vi "DTM Receiver Test.vi"() -> ()   [LabVIEW 2026, in "Nordic nRF52 DK DTM Test.lvlib"]
uses:
  Nordic nRF52 DK DTM Test.lvlib
  <vilib>/Analysis/1siggen.llb/Ramp Pattern by Delta.vi
  <vilib>/Analysis/NI_AALBase.lvlib
panel:
  in  "stop":bool
  out "Waveform Chart":T1(graph)
  out "iteration":i32
  out "Packets Received":u16
  out "Current Power":dbl
  out "Receiver Sensitivity, dBm":dbl
  in  "Baud Rate":u32=19200
  in  "Com Port Resource":refnum<visa-resource-name>="COM3"
  in  "Power Step, dBm":dbl=-0.2
  in  "Power Stop, dBm":dbl=-100.0
  in  "Power Start, dBm":dbl=-70.0
  in  "BLE Channel (0-39)":u8=19 max=39 step=1
  out "Rx Sens Threshold":i32
  in  "Packets to Generate":i32=1500
  in  "BLE Waveform Path":path=path "C:/git/LabVIEW_Bluetooth_Examples/BLE DTM Test/Waveform Files/BLE_PRBS9.tdms"
  in  "External Attenuation (dB)":dbl=1.1
  in  "Reference Clock Source":string(combo)="OnboardClock"
  in  "RFSG Resource":refnum<k15>="VST" caption="resource name"
  out "error out":errorcluster
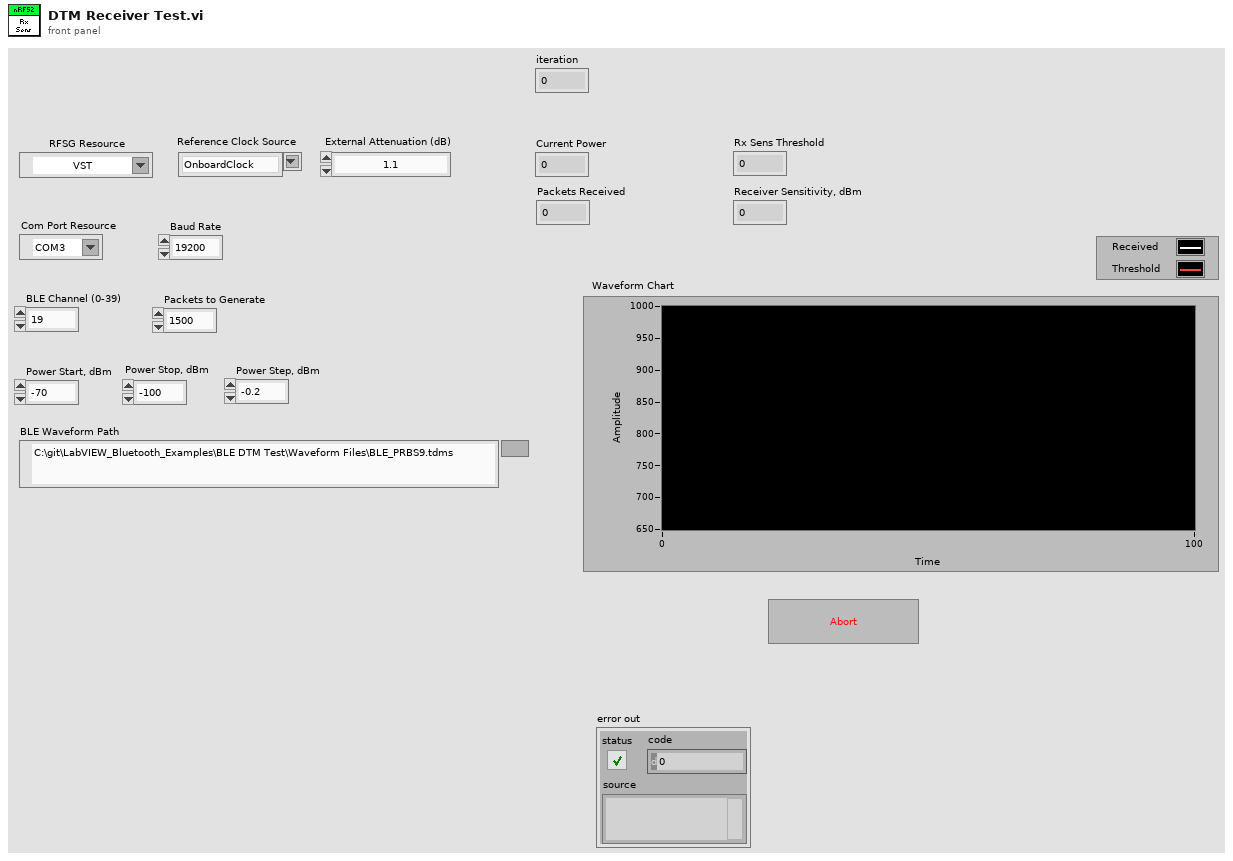
[diagram p1: front panel]
types:
  T1 = cluster{"Returned Packet Count":u16, "Rx Sensitivity Threshold":i32}
  T2 = cluster{"Returned Packet Count":u16, "Rx Sensitivity Threshold":i32}[]
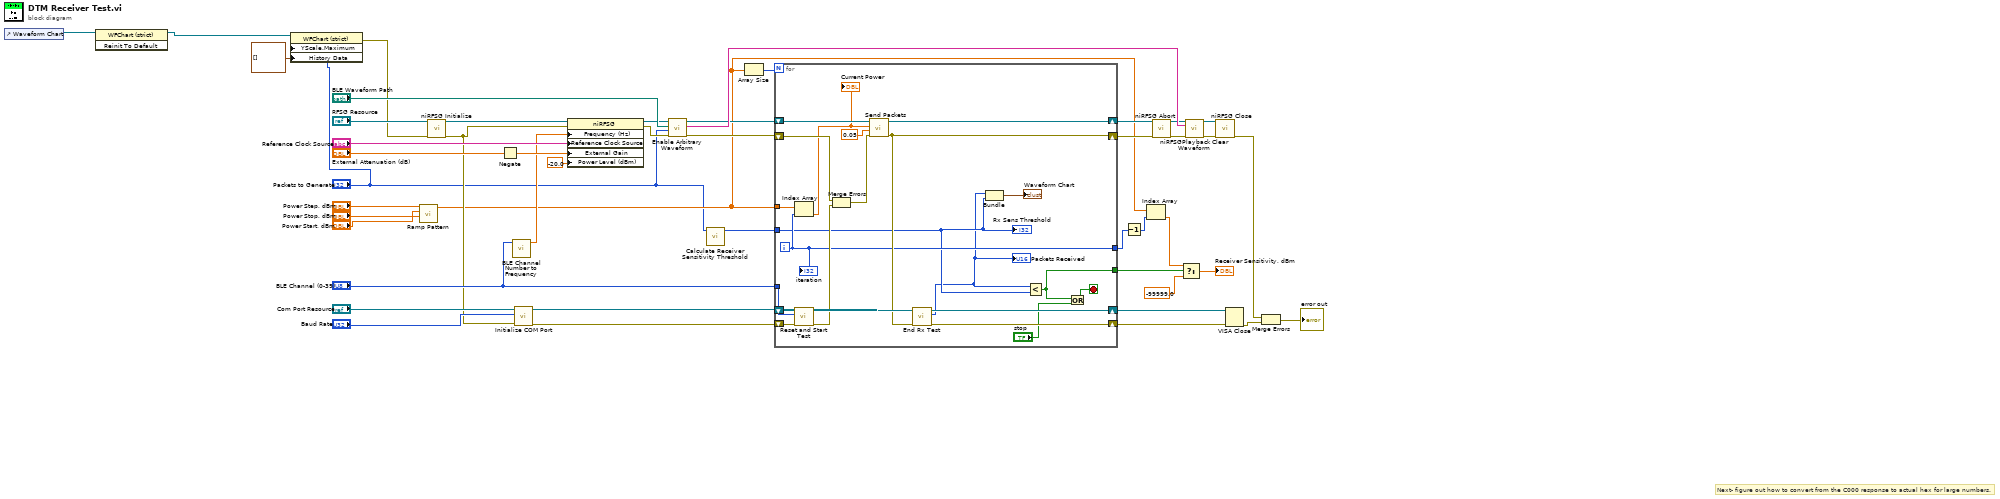
[diagram p0: block diagram]
diagram:
  # "Next- figure out how to convert from the C000 response to actual hex for large numbers."
  n1 = control-ref of="Waveform Chart"() -> (w5:refnum<vi>)
  n2 = invoke class="WFChart (strict)" method="Reinit To Default"(reference=w5) -> (reference out=w4:refnum<vi>)  [unwired: 2 in, 2 out]
  n3 = property class="WFChart (strict)"(reference=w4, "YScale.Maximum"="Packets to Generate", "History Data"=T2 []) -> (error out=w3:errorcluster)  [unwired: 1 in, 1 out]
  n4 = call-poly <vilib>:"Ramp Pattern.vi"("start"="Power Start, dBm", "end"="Power Stop, dBm", "delta"="Power Step, dBm") -> ("Ramp Pattern"=w6:dbl[])  [unwired: 6 in, 2 out]
  n5 = call <instrlib>:"niRFSG Initialize.vi"("resource name"="RFSG Resource", "error in"=w3) -> ("instrument handle"=w36:refnum<k15>, "error out"=w15:errorcluster)  [unwired: 2 in, 10 out]
  n6 = Negate(x="External Attenuation (dB)") -> (-x=w34:dbl)
  n7 = call "BLE Channel Number to Frequency.vi"("BLE  Channel"="BLE Channel (0-39)") -> ("Frequency, Hz"=w27:dbl)  [unwired: 9 in, 1 out]
  n8 = call "Initialize COM Port.vi"("error in (no error)"=w15, "baud rate (9600)"="Baud Rate", "VISA Refnum in"="Com Port Resource") -> ("error out"=w46:errorcluster, "VISA Refnum out"=w45:refnum<visa-resource-name>)  [unwired: 7 in]
  n9 = property class="niRFSG"(reference=w36, error in=w15, "Frequency (Hz)"=w27, "Reference Clock Source"="Reference Clock Source", "External Gain"=w34, "Power Level (dBm)"=-20.0 ("RF:Power Level (dBm)")) -> (reference out=w28:refnum<k15>, error out=w29:errorcluster)
  n10 = call "Enable Arbitrary Waveform.vi"("error in (no error)"=w29, "Packets to Generate"="Packets to Generate", "BLE Waveform Path"="BLE Waveform Path", "IVI Refnum in"=w28) -> ("error out"=w20:errorcluster, "waveform name"=w32:string, "IVI Refnum out"=w21:refnum<k15>)  [unwired: 5 in]
  n11 = call "Calculate Receiver Sensitivity Threshold.vi"("Packets to Generate"="Packets to Generate") -> ("Rx Sensitivity Threshold"=w14:i32)  [unwired: 10 in]
  n12 = Array Size(array=w6) -> (size(s)=w7:i32)
  n13 = for {
    N: w7 -> [_]
    shift-right: [w65] -> w39
    shift-left: w46 -> [w59]
    shift-right: [w67] -> w42
    shift-left: w45 -> [w69]
    shift-right: [w63] -> w31
    shift-left: w21 -> [w61]
    shift-right: [w62] -> w30
    shift-left: w20 -> [w64]
    tunnel: w6 -> [w56]
    tunnel: "BLE Channel (0-39)" -> [w60]
    tunnel: w14 -> [w53]
    tunnel: [w55] -> w13
    tunnel: [w50] -> w11
    i -> [w55]
    stop <- w49 stop-if-true
    n14 = Index Array(array=w56, index=w55) -> (element=w54:dbl)
    "Current Power" <- w54
    n15 = call "Reset and Start Test.vi"("error in (no error)"=w59, "BLE Channel Number (0-39)"=w60, "VISA Refnum in"=w69) -> ("error out"=w66:errorcluster, "VISA Refnum out"=w68:refnum<visa-resource-name>)  [unwired: 6 in, 1 out]
    n16 = Merge Errors(w64, w66) -> (w58:errorcluster)
    n17 = call "Send Packets.vi"("error in (no error)"=w58, "Delay before packets, sec"=0.05 ("Delay before packets"), "SG Power, dBm"=w54, "IVI Refnum in"=w61) -> ("error out"=w62:errorcluster, "IVI Refnum out"=w63:refnum<k15>)  [unwired: 6 in]
    n18 = call "End Rx Test.vi"("error in (no error)"=w62, "VISA Refnum in"=w68) -> ("error out"=w65:errorcluster, "Returned Packet Count"=w52:u16, "VISA Refnum out"=w67:refnum<visa-resource-name>)  [unwired: 7 in]
    "Packets Received" <- w52
    n19 = Bundle("Returned Packet Count"=w52, "Rx Sensitivity Threshold"=w53) -> (→"Waveform Chart":T1)  [unwired: 1 in]
    n20 = Less?(x=w52, y=w53) -> (x < y?=w50:bool)
    n21 = Or(x=w50, y="stop") -> (x .or. y?=w49:bool)
    "Rx Sens Threshold" <- w53
    "iteration" <- w55
  }
  n22 = Decrement(x=w13) -> (x-1=w12:i32)
  n23 = Index Array(array=w6, index=w12) -> (element=w10:dbl)
  n24 = call <instrlib>:"niRFSG Abort.vi"("instrument handle"=w31, "error in"=w30) -> ("instrument handle out"=w16:refnum<k15>, "error out"=w17:errorcluster)  [unwired: 12 out]
  n25 = Select(t=w10, s=w11, f=-99999.0) -> (s? t:f=→"Receiver Sensitivity, dBm":dbl)
  n26 = call <instrlib>:"niRFSGPlayback Clear Waveform.vi"("instrument handle in"=w16, "waveform name"=w32, "error in"=w17) -> ("instrument handle out"=w18:refnum<k15>, "error out"=w19:errorcluster)  [unwired: 11 in]
  n27 = call <instrlib>:"niRFSG Close.vi"("instrument handle"=w18, "error in"=w19) -> ("error out"=w37:errorcluster)  [unwired: 13 out]
  n28 = VISA Close(VISA resource name=w42, error in (no error)=w39) -> (error out=w43:errorcluster)
  n29 = Merge Errors(w37, w43) -> (→"error out":errorcluster)
